vi "Module - SQL Client.vi"(8 "error in (no error)":errorcluster) -> (0 "error out":errorcluster)   [LabVIEW 2020]
uses:
  Control/State - SQL Client.ctl
  Control/Data Type - OPC to SQL.ctl
  Control/State - eFGV.ctl
  SubVI/Database/Control/mysql_authentication.ctl
  Control/Config File Selection.ctl
  Control/Cluster - SQL Reply.ctl
panel:
  out "2D String":string[][](array[string])
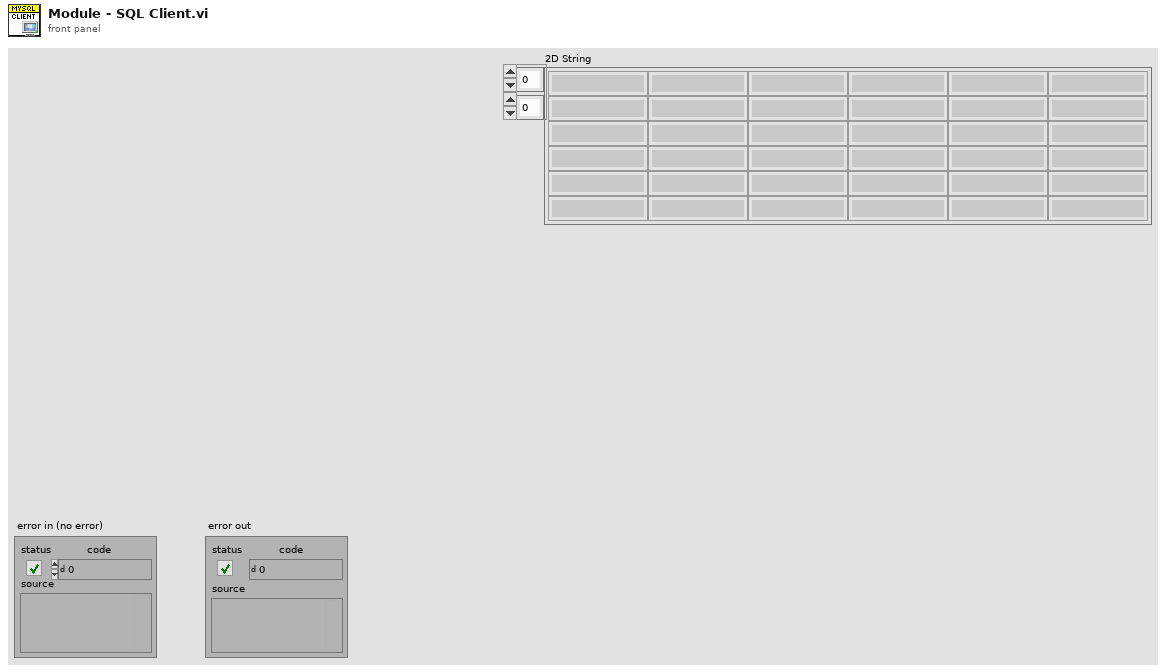
[diagram p1: front panel]
types:
  T1 = typedef "Data Type - OPC to SQL.ctl" = cluster{"DB Message":string, "DB Command":string, "Module Name":string}
  T2 = cluster{"TOut":i32, "Data Type - OPC to SQL":T1, "SQL Reply":string[][], "SQL Refnum":refnum<k5>, "User Exit":bool, "SQL Connected":bool}
  T3 = typedef "State - SQL Client.ctl" = enum16{"Init module", "Register for event", "Idle", "Connect to SQL Server", "Send query to SQL", "Send reply to eFGV", "Disconnect from SQL Server", "Unregister user event", "Close module"}
  T4 = typedef "Config File Selection.ctl" = enum16{"Modbus", "SQL", "General"}
  T5 = typedef "mysql_authentication.ctl" = cluster{"User":string, "Password":string, "Database":string}
  T6 = typedef "State - eFGV.ctl" = enum16{"Init", "Read", "Write", "Close"}
  T7 = typedef "Cluster - SQL Reply.ctl" = cluster{"DB Message":string, "Module Name":string, "Reply Data":string[][]}
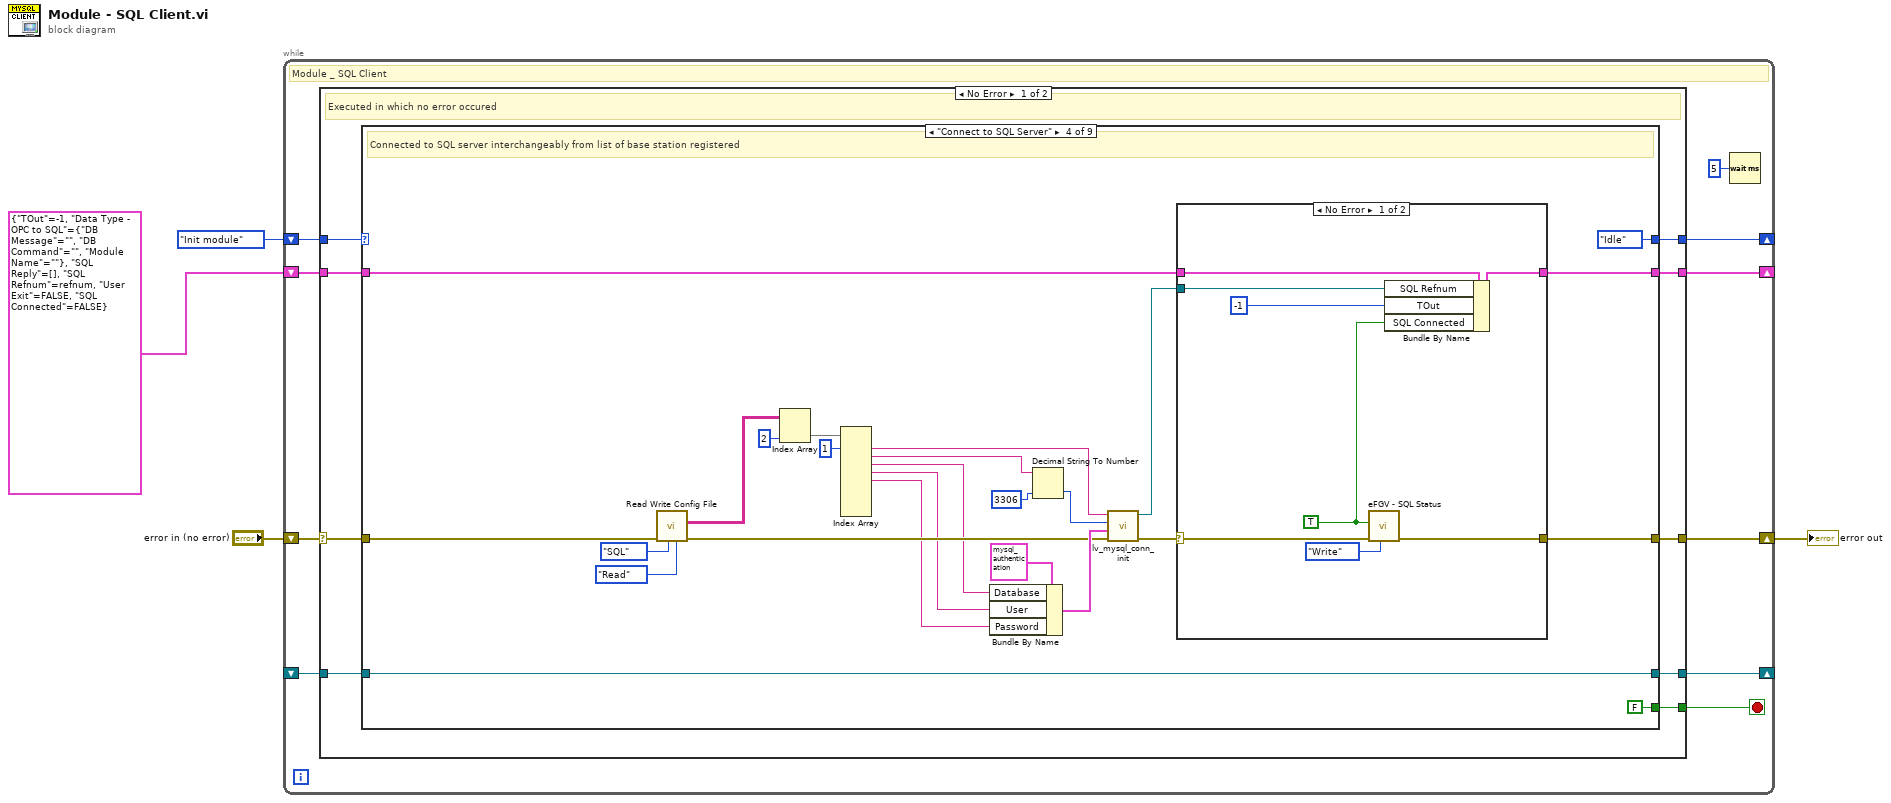
[diagram p0: block diagram]
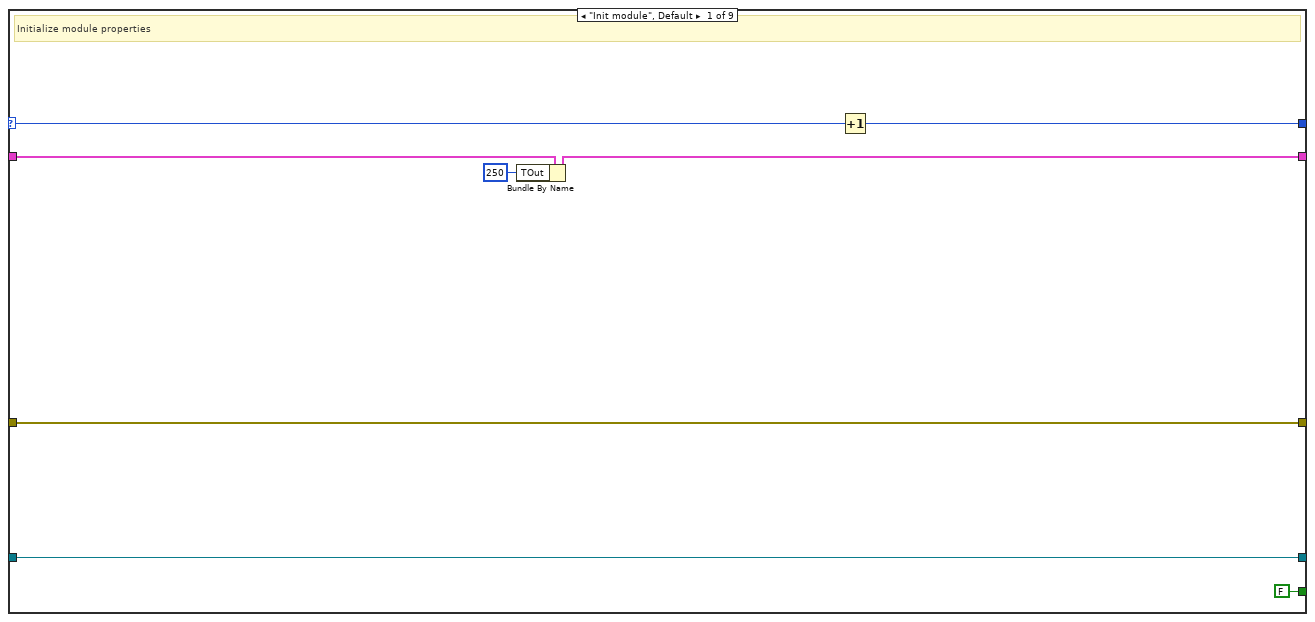
[diagram p2: hidden frame]
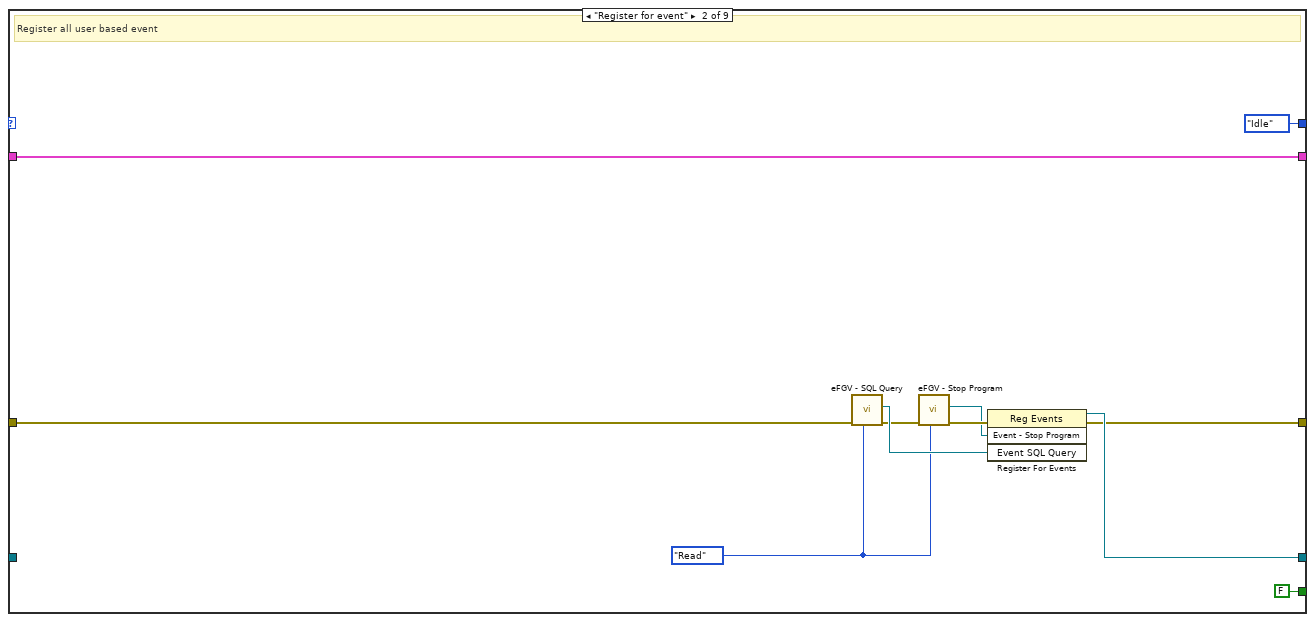
[diagram p3: hidden frame]
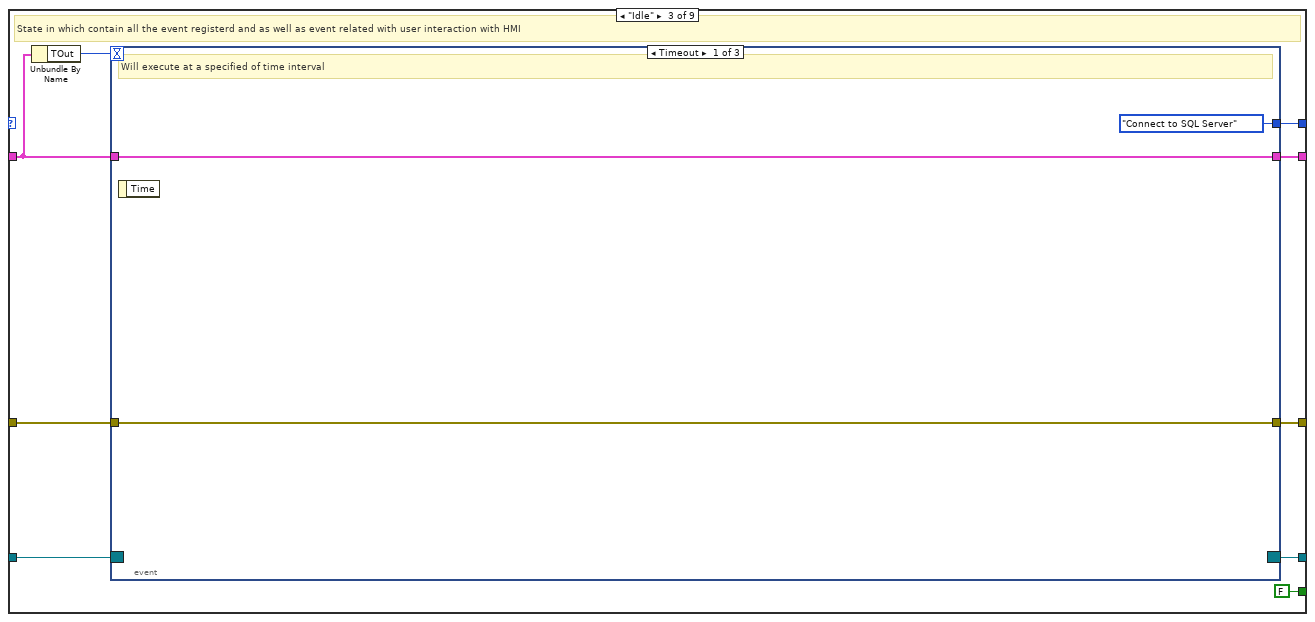
[diagram p4: hidden frame]
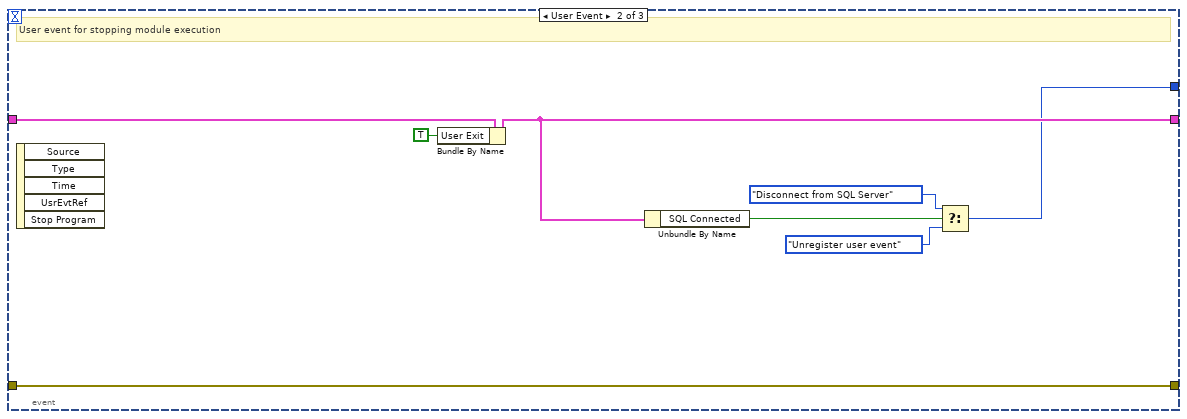
[diagram p5: hidden frame]
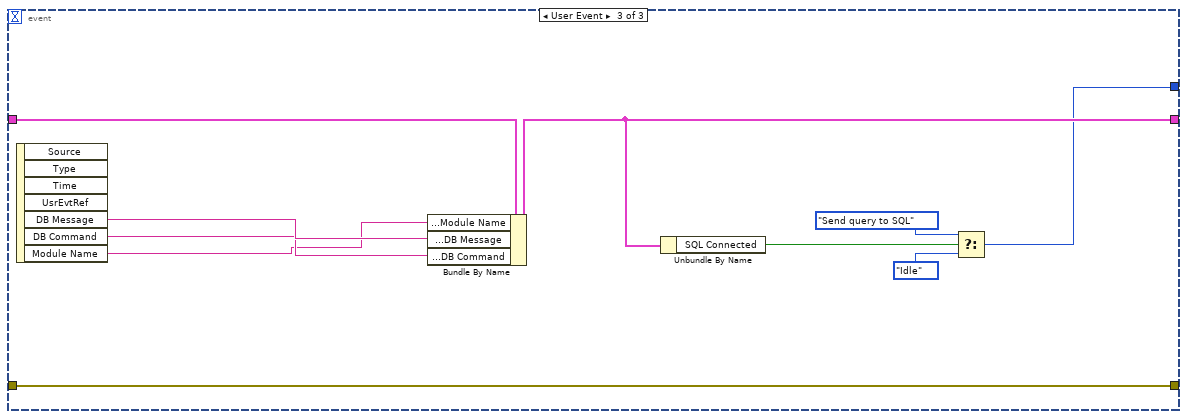
[diagram p6: hidden frame]
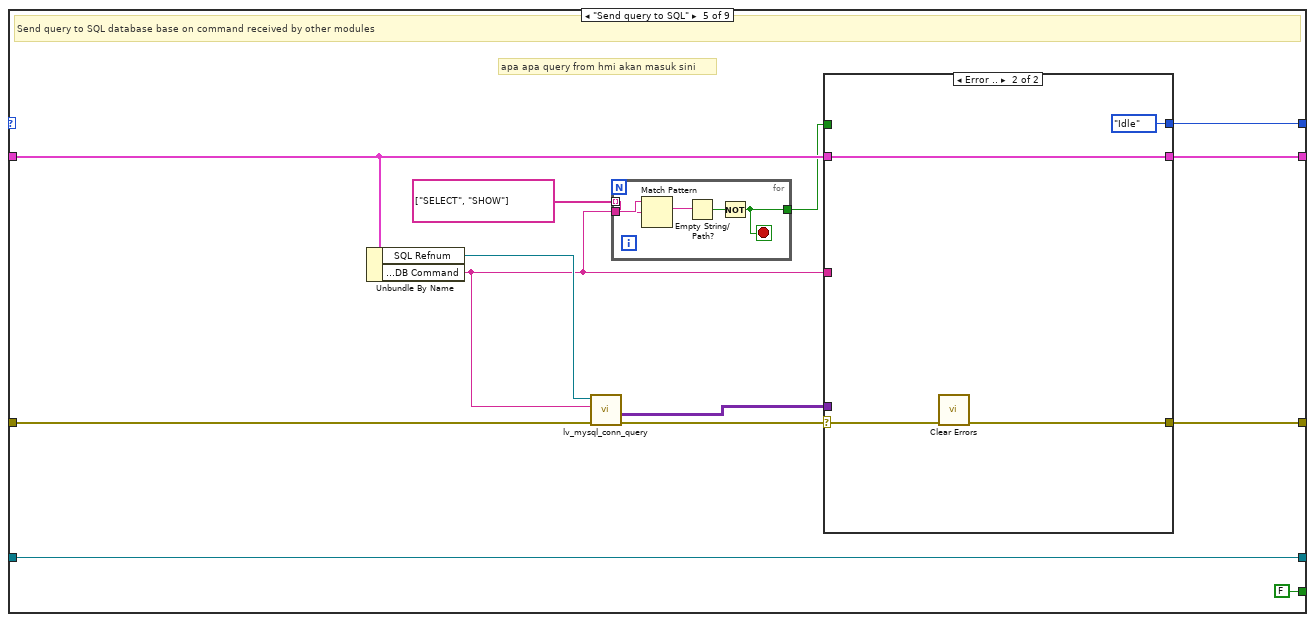
[diagram p8: hidden frame]
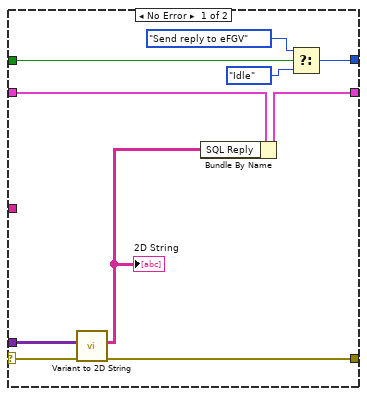
[diagram p9: hidden frame]
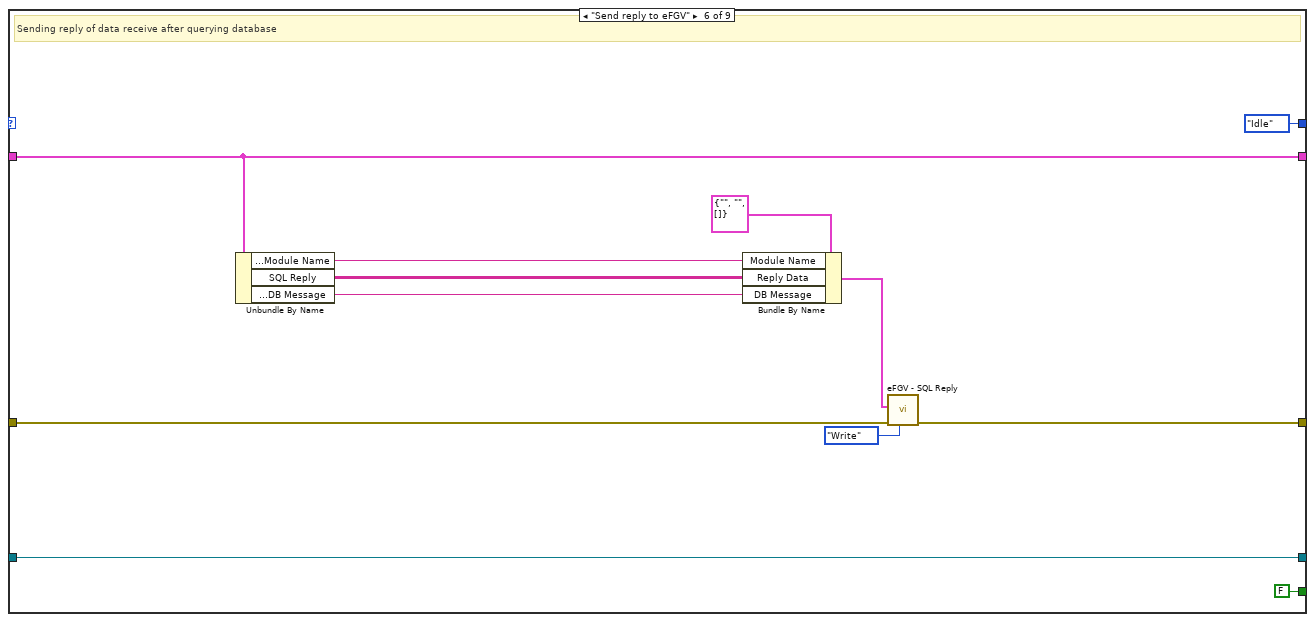
[diagram p10: hidden frame]
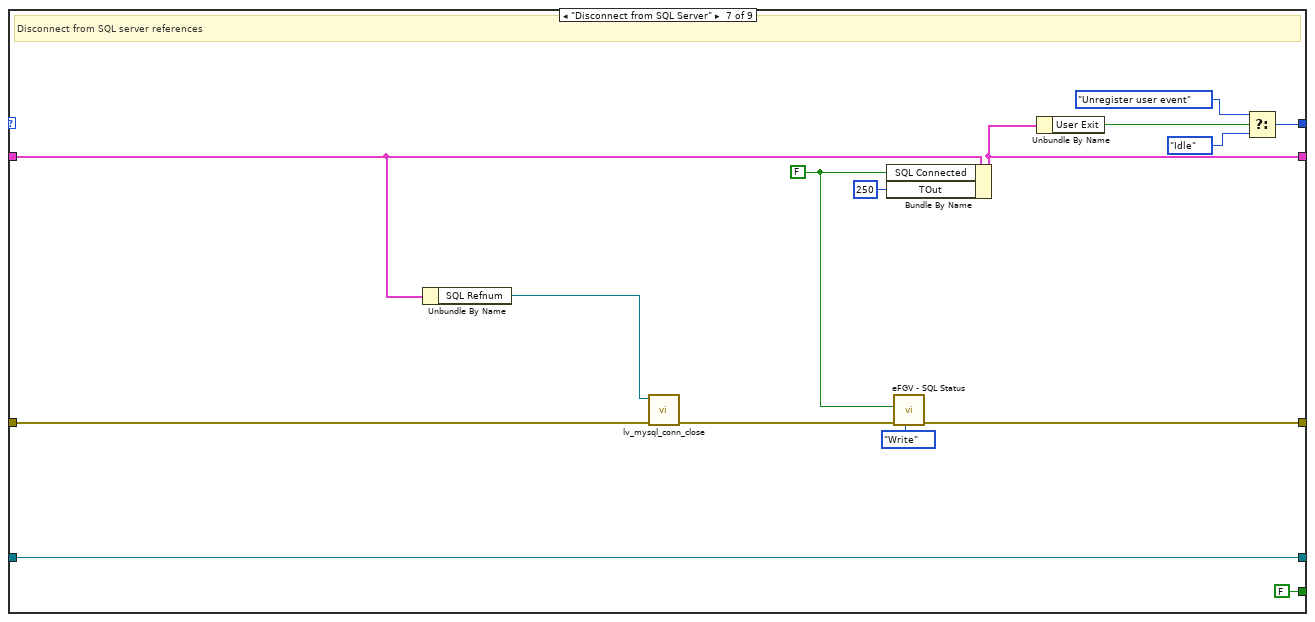
[diagram p11: hidden frame]
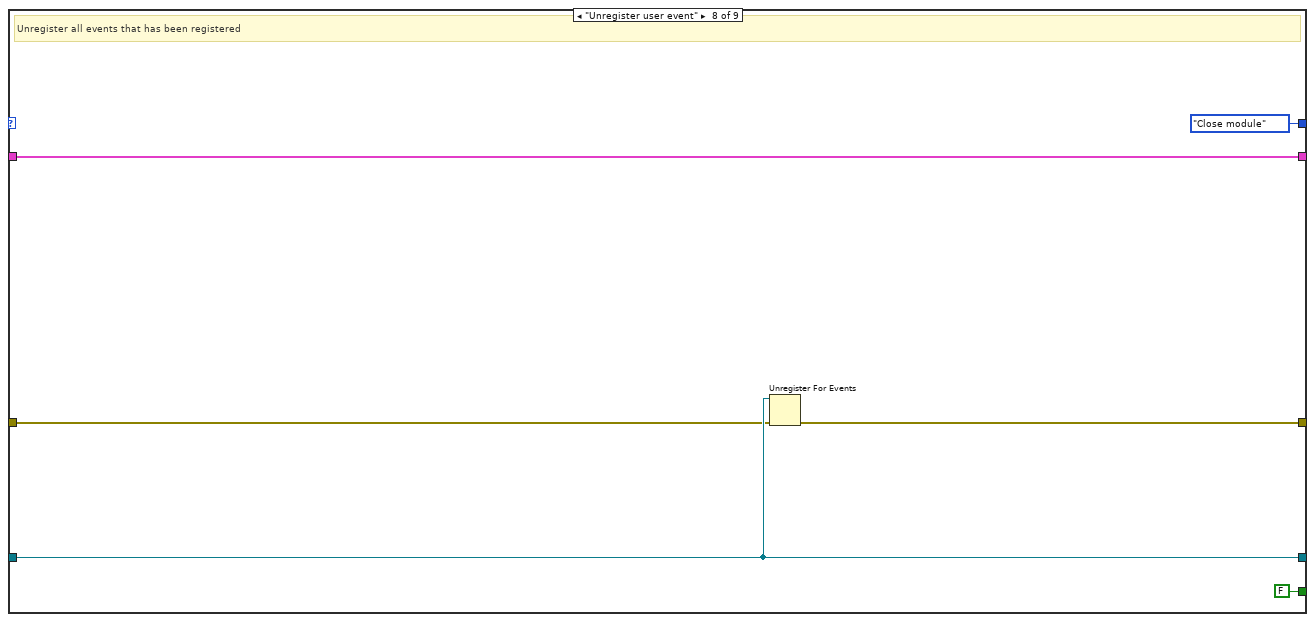
[diagram p12: hidden frame]
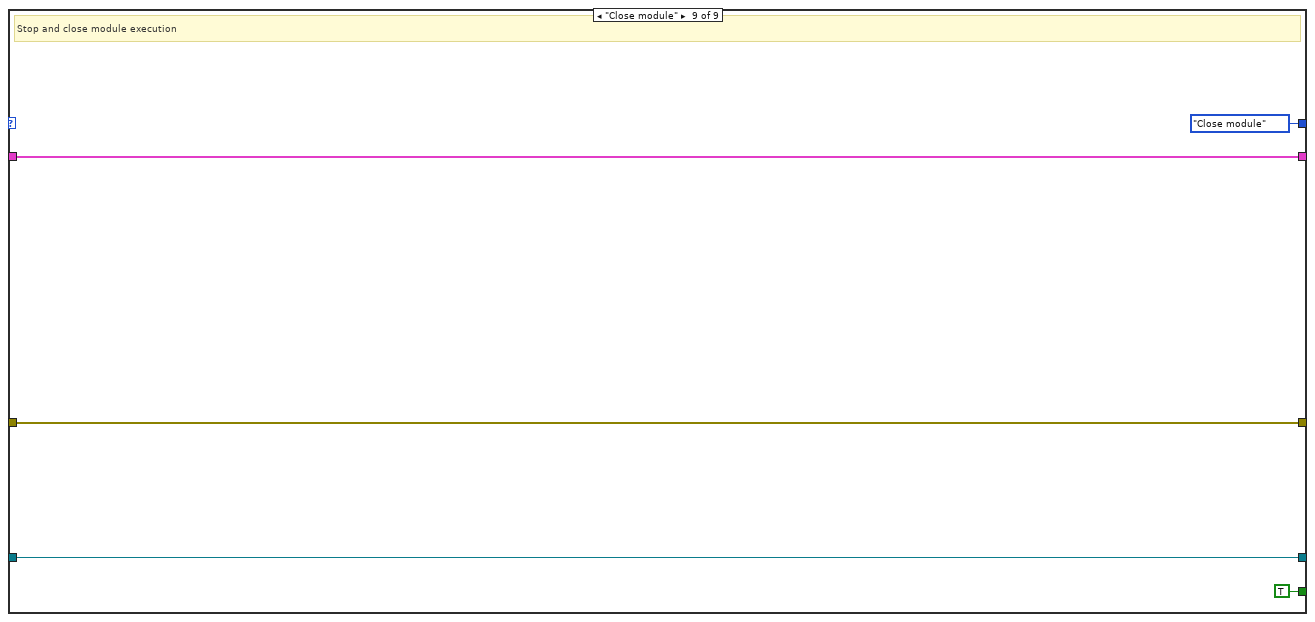
[diagram p13: hidden frame]
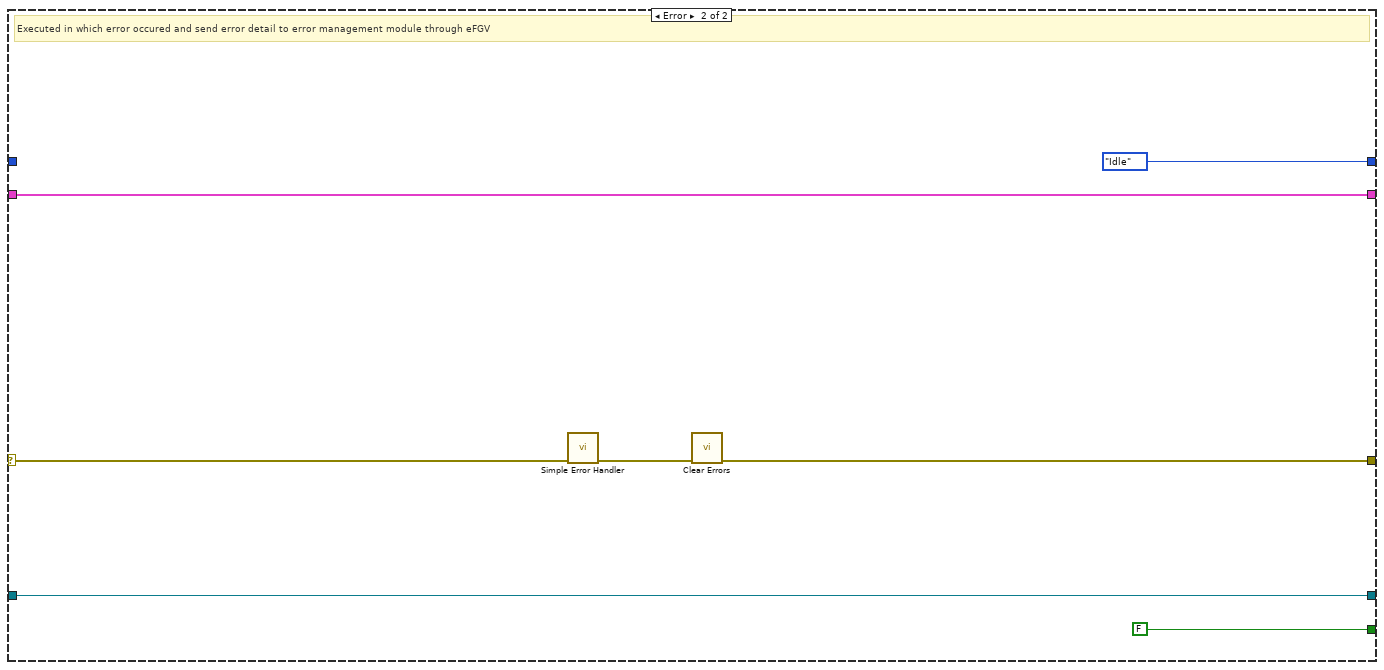
[diagram p14: hidden frame]
diagram:
  n1 = while {
    shift-right: [w10] -> w3
    shift-left: "error in (no error)" -> [w14]
    shift-right: [w6] -> _
    shift-left: State_-_SQL_Client."Init module" -> [w12]
    shift-right: [w9] -> _
    shift-left: T2 {"TOut"=-1, "Data Type - OPC to SQL"={"DB Message"="", "DB Command"="", "Module Name"=""}, "SQL Reply"=[], "SQL Refnum"=refnum, "User Exit"=FALSE, "SQL Connected"=FALSE} -> [w11]
    shift-right: [w8] -> _
    shift-left: _ -> [w7]
    stop <- w13 stop-if-true
    # "Module _ SQL Client"
    n2 = case shown="No Error" w14 {
      selector: w14 -> [w23 w182]
      tunnel: [w22 FALSE] -> w13
      tunnel: w12 -> [w15 _]
      tunnel: w11 -> [w21 w179]
      tunnel: [w20 w180] -> w10
      tunnel: [w19 w179] -> w9
      tunnel: [w18 w183] -> w8
      tunnel: w7 -> [w17 w183]
      tunnel: [w16 State_-_SQL_Client."Idle"] -> w6
      frame No Error {
        # "Executed in which no error occured"
        n3 = case shown="\"Connect to SQL Server\"" w15 {
          selector: w15 -> [w25 _ _ _ _ _ _ _ _]
          tunnel: w23 -> [w26 w36 w49 w85 w117 w149 w164 w168 w177]
          tunnel: [FALSE FALSE FALSE FALSE FALSE FALSE FALSE FALSE TRUE] -> w22
          tunnel: w21 -> [w30 w40 w46 w94 w116 w147 w160 w167 w176]
          tunnel: [w26 w37 w48 w92 w113 w148 w157 w172 w177] -> w20
          tunnel: [w28 w40 w45 w91 w114 w147 w155 w167 w176] -> w19
          tunnel: [w29 w41 w50 w97 w120 w151 w166 w171 w175] -> w18
          tunnel: w17 -> [w29 _ w51 w97 w120 w151 w166 w171 w175]
          tunnel: [w24 State_-_SQL_Client."Idle" w43 State_-_SQL_Client."Idle" w119 State_-_SQL_Client."Idle" w163 State_-_SQL_Client."Close module" State_-_SQL_Client."Close module"] -> w16
          frame "Init module", Default {
            # "Initialize module properties"
            n4 = Bundle By Name(cluster=w30, "TOut"=250) -> (w28:T2)
            n5 = Increment(x=w25) -> (x+1=w24:T3)
          }
          frame "Register for event" {
            w32 = State_-_eFGV."Read" ("State")
            # "Register all user based event"
            n6 = call "eFGV - SQL Query.vi"("State"=w32, "error in (no error)"=w36) -> ("error out"=w34:errorcluster, "Event SQL Query"=w39:refnum<user-event>)  [unwired: 8 in]
            n7 = call "eFGV - Stop Program.vi"("State - eFGV"=w32, "error in (no error)"=w34) -> ("error out"=w35:errorcluster, "Event - Stop Program"=w33:refnum<user-event>)  [unwired: 8 in]
            n8 = register-events(error in=w35, w33, w39) -> (reference out=w41:refnum<event-registration>, error out=w37:errorcluster)  [unwired: 1 in]
          }
          frame "Idle" {
            # "State in which contain all the event registerd and as well as event related with user interaction with HMI"
            n9 = Unbundle By Name(w46) -> ("TOut"=w47:i32)
            n10 = event shown="[0] Timeout" {
              selector: w51 -> [_ _ _]
              dyn-events: [_ _ _] -> w50
              timeout: w47 -> [_ _ _]
              tunnel: w49 -> [w54 w61 w64]
              tunnel: [w54 w61 w64] -> w48
              tunnel: w46 -> [w53 w62 w67]
              tunnel: [w53 w57 w66] -> w45
              tunnel: [State_-_SQL_Client."Connect to SQL Server" w55 w65] -> w43
              event Timeout {
                # "Will execute at a specified of time interval"
                n11 = event-data() -> ()  [unwired: 1 in, 1 out]
              }
              event User Event {
                # "User event for stopping module execution"
                n12 = event-data() -> ()  [unwired: 1 in, 5 out]
                n13 = Bundle By Name(cluster=w62, "User Exit"=TRUE) -> (w57:T2)
                n14 = Unbundle By Name(w57) -> ("SQL Connected"=w56:bool)
                n15 = Select(t=State_-_SQL_Client."Disconnect from SQL Server", s=w56, f=State_-_SQL_Client."Unregister user event") -> (s? t:f=w55:T3)
              }
              event User Event {
                n16 = event-data() -> ("DB Message"=w69:string, "DB Command"=w68:string, "Module Name"=w63:string)  [unwired: 1 in, 4 out]
                n17 = Bundle By Name(cluster=w67, "Data Type - OPC to SQL.Module Name"=w63, "Data Type - OPC to SQL.DB Message"=w69, "Data Type - OPC to SQL.DB Command"=w68) -> (w66:T2)
                n18 = Unbundle By Name(w66) -> ("SQL Connected"=w72:bool)
                n19 = Select(t=State_-_SQL_Client."Send query to SQL", s=w72, f=State_-_SQL_Client."Idle") -> (s? t:f=w65:T3)
              }
            }
          }
          frame "Connect to SQL Server" {
            # "Connected to SQL server interchangeably from list of base station registered"
            n20 = call "Read Write Config File.vi"("Operation"=enum16{"Read", "Write"}."Read", "Config File"=Config_File_Selection."SQL", "error in (no error)"=w85) -> ("error out"=w84:errorcluster, "Section-Key-Value Out"=w81:string[][])  [unwired: 7 in]
            n21 = Index Array(array=w81, index (col)=2 ("disabled index (col)")) -> (element=w79:string[])  [unwired: 1 in]
            n22 = Index Array(array=w79, index #1=1 ("index")) -> (element #1=w77:string, element #2=w76:string, element #3=w75:string, element #4=w74:string, element #5=w73:string)  [unwired: 8 in, 4 out]
            n23 = Bundle By Name(cluster=T5 {"User"="VSysOEE", "Password"="Visinergy@123", "Database"="vsys_oee"} ("Authentication"), "Database"=w75, "User"=w74, "Password"=w73) -> (w86:T5)
            n24 = Decimal String To Number(string=w76, default (0L)=u16 3306 ("Port")) -> (number=w88:u16)  [unwired: 1 in, 1 out]
            n25 = call "lv_mysql_conn_init.vi"("error in (no error)"=w84, "Authentication"=w86, "Port"=w88, "IP Address"=w77) -> ("error out"=w93:errorcluster, "connection ID out"=w90:refnum<k5>)  [unwired: 6 in]
            n26 = case shown="No Error" w93 {
              selector: w93 -> [w101 w106]
              tunnel: w94 -> [w105 w107]
              tunnel: [w100 w106] -> w92
              tunnel: [w104 w107] -> w91
              tunnel: w90 -> [w103 _]
              frame No Error {
                w98 = TRUE ("SQL Connected")
                n27 = call "eFGV - SQL Status.vi"("State"=State_-_eFGV."Write", "error in (no error)"=w101, "SQL Connected"=w98) -> ("error out"=w100:errorcluster)  [unwired: 7 in, 1 out]
                n28 = Bundle By Name(cluster=w105, "SQL Refnum"=w103, "TOut"=-1, "SQL Connected"=w98) -> (w104:T2)
              }
              frame Error {
              }
            }
          }
          frame "Send query to SQL" {
            # "apa apa query from hmi akan masuk sini"
            # "Send query to SQL database base on command received by other modules"
            n29 = Unbundle By Name(w116) -> ("SQL Refnum"=w115:refnum<k5>, "Data Type - OPC to SQL.DB Command"=w108:string)
            n30 = call "lv_mysql_conn_query.vi"("error in (no error)"=w117, "Query"=w108, "connection ID"=w115) -> ("error out"=w111:errorcluster, "Return Data"=w112:variant[][])  [unwired: 5 in, 2 out]
            n31 = for {
              tunnel: w108 -> [w124]
              tunnel: [w121] -> w110
              tunnel: string[] ["SELECT", "SHOW"] -> [w123] mode=indexing
              stop <- w121 stop-if-true
              n32 = Match Pattern(string=w124, regular expression=w123) -> (match substring=w125:string)  [unwired: 1 in, 3 out]
              n33 = Empty String/Path?(string/path=w125) -> (empty?=w122:bool)
              n34 = Not(x=w122) -> (.not. x?=w121:bool)
            }
            n35 = case shown="Error .." w111 {
              selector: w111 -> [w131 w137]
              tunnel: [w129 State_-_SQL_Client."Idle"] -> w119
              tunnel: w116 -> [w135 w138]
              tunnel: [w134 w138] -> w114
              tunnel: [w133 w136] -> w113
              tunnel: w112 -> [w132 _]
              tunnel: w108 -> [_ _]
              tunnel: w110 -> [w128 _]
              frame No Error {
                n36 = call "Variant to 2D String.vi"("error in (no error)"=w131, "Variant"=w132) -> ("error out"=w133:errorcluster, "2D String"=w126:string[][])  [unwired: 8 in]
                "2D String" <- w126
                n37 = Bundle By Name(cluster=w135, "SQL Reply"=w126) -> (w134:T2)
                n38 = Select(t=State_-_SQL_Client."Send reply to eFGV", s=w128, f=State_-_SQL_Client."Idle") -> (s? t:f=w129:T3)
              }
              frame Error {
                n39 = call <vilib>:"Clear Errors.vi"("error in (no error)"=w137) -> ("error out"=w136:errorcluster)  [unwired: 5 in, 1 out]
              }
            }
          }
          frame "Send reply to eFGV" {
            # "Sending reply of data receive after querying database"
            n40 = Unbundle By Name(w147) -> ("Data Type - OPC to SQL.Module Name"=w144:string, "SQL Reply"=w145:string[][], "Data Type - OPC to SQL.DB Message"=w140:string)
            n41 = Bundle By Name(cluster=T7 {"DB Message"="", "Module Name"="", "Reply Data"=[]} ("SQL Reply"), "Module Name"=w144, "Reply Data"=w145, "DB Message"=w140) -> (w141:T7)
            n42 = call "eFGV - SQL Reply.vi"("State"=State_-_eFGV."Write", "error in (no error)"=w149, "SQL Reply"=w141) -> ("error out"=w148:errorcluster)  [unwired: 7 in, 1 out]
          }
          frame "Disconnect from SQL Server" {
            w154 = FALSE ("SQL Connected")
            # "Disconnect from SQL server references"
            n43 = Unbundle By Name(w160) -> ("SQL Refnum"=w152:refnum<k5>)
            n44 = call "lv_mysql_conn_close.vi"("error in (no error)"=w164, "connection ID"=w152) -> ("error out"=w158:errorcluster)  [unwired: 9 in]
            n45 = Bundle By Name(cluster=w160, "SQL Connected"=w154, "TOut"=250) -> (w155:T2)
            n46 = call "eFGV - SQL Status.vi"("State"=State_-_eFGV."Write", "error in (no error)"=w158, "SQL Connected"=w154) -> ("error out"=w157:errorcluster)  [unwired: 7 in, 1 out]
            n47 = Unbundle By Name(w155) -> ("User Exit"=w159:bool)
            n48 = Select(t=State_-_SQL_Client."Unregister user event", s=w159, f=State_-_SQL_Client."Idle") -> (s? t:f=w163:T3)
          }
          frame "Unregister user event" {
            # "Unregister all events that has been registered"
            n49 = Unregister For Events(event registration refnum=w171, error in=w168) -> (error out=w172:errorcluster)
          }
          frame "Close module" {
            # "Stop and close module execution"
          }
        }
      }
      frame Error {
        # "Executed in which error occured and send error detail to error management module through eFGV"
        n50 = call <vilib>:"Simple Error Handler.vi"("error in (no error)"=w182) -> ("error out"=w181:errorcluster)  [unwired: 4 in, 4 out]
        n51 = call <vilib>:"Clear Errors.vi"("error in (no error)"=w181) -> ("error out"=w180:errorcluster)  [unwired: 5 in, 1 out]
      }
    }
    n52 = Wait (ms)(milliseconds to wait=u32 5) -> ()  [unwired: 1 out]
  }
  "error out" <- w3
